vi "Destroy Helper Loop Events.vi"(11 "Acquisition UI in":refnum<class "Acquisition UI.lvclass">) -> ()   [LabVIEW 2018, in "Acquisition UI.lvlib" / "Acquisition UI.lvclass"]
uses:
  Acquisition UI.lvclass
  Acquisition UI.lvclass/Acquisition UI.ctl
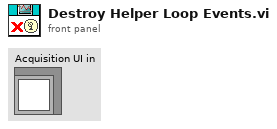
[diagram p1: front panel]
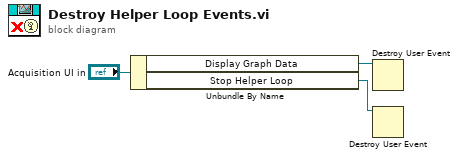
[diagram p0: block diagram]
diagram:
  n1 = Unbundle By Name("Acquisition UI in") -> ("Display Graph Data"=w2:refnum<user-event>, "Stop Helper Loop"=w3:refnum<user-event>)
  n2 = Destroy User Event(user event=w2) -> ()  [unwired: 1 in, 1 out]
  n3 = Destroy User Event(user event=w3) -> ()  [unwired: 1 in, 1 out]
